vi "SVN Master Method Checkout.vi"(8 "error in (no error)":errorcluster, 11 "Method Name":string) -> (0 "error out":errorcluster, 1 "Method Version":i32, 2 "versions":i32[](array[numeric]), 3 "Method Names":string[](array[string]), 4 "Method Exists":bool, 6 "method version folder":path)   [LabVIEW 2012]
uses:
  Folders.ctl
  ReadWrite.ctl
  Which method type.ctl
  Design Server.lvlib
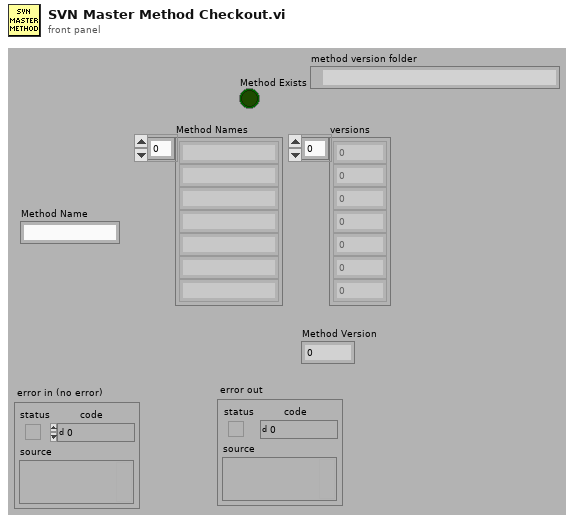
[diagram p1: front panel]
types:
  T1 = typedef "Design Server.lvlib/Folders.ctl" = enum16{"MathcadMethods", "RequestedDesigns", "CompletedDesigns", "MathcadCode", "CollabnetSVN.exe"}
  T2 = typedef "ReadWrite.ctl" = enum16{"Read", "Write"}
  T3 = typedef "Which method type.ctl" = enum16{"Master Method", "Method"}
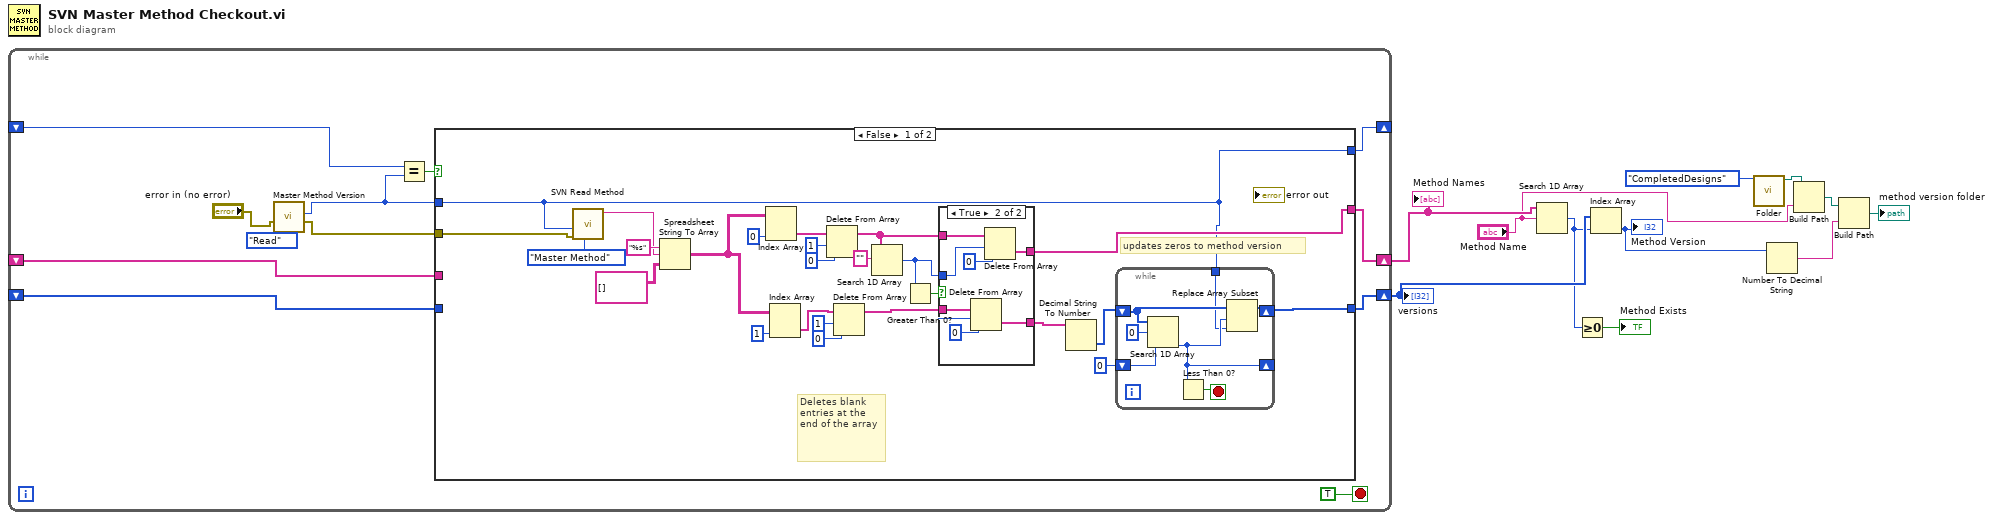
[diagram p0: block diagram]
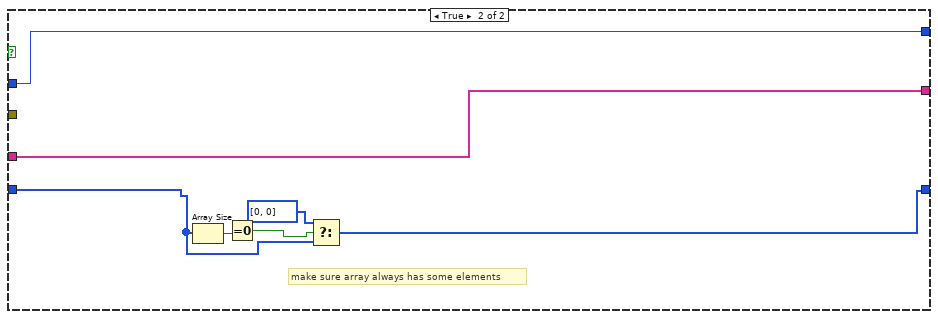
[diagram p3: hidden frame]
diagram:
  n1 = while {
    shift-right: [w20] -> _
    shift-left: _ -> [w22]
    shift-right: [w19] -> w11
    shift-left: _ -> [w17]
    shift-right: [w18] -> w10
    shift-left: _ -> [w16]
    stop <- TRUE stop-if-true
    n2 = call "Master Method Version.vi"("Config"=ReadWrite."Read", "error in (no error)"="error in (no error)") -> ("error out"=w13:errorcluster, "Current Master Method Version"=w12:i32)  [unwired: 6 in, 2 out]
    n3 = Equal?(x=w22, y=w12) -> (x = y?=w21:bool)
    n4 = case shown="False" w21 {
      tunnel: w12 -> [w25 w70]
      tunnel: [w25 w70] -> w20
      tunnel: [w27 w65] -> w18
      tunnel: [w26 w71] -> w19
      tunnel: w17 -> [_ w71]
      tunnel: w16 -> [_ w66]
      tunnel: w13 -> [w24 _]
      frame False {
        # "updates zeros to method version"
        # "Deletes blank entries at the end of the array"
        n5 = call "SVN Read Method.vi"("Which Method Type"=Which_method_type."Master Method", "error in (no error)"=w24, "Method version"=w25) -> ("Method text"=w29:string)  [unwired: 6 in, 2 out]
        n6 = Spreadsheet String To Array(format string="%s", spreadsheet string=w29, array type (2D Dbl)=string[][] []) -> (array=w34:string[][])  [unwired: 1 in]
        n7 = Index Array(array=w34, index (col)=0 ("index")) -> (element=w43:string[])  [unwired: 1 in]
        n8 = Index Array(array=w34, index (col)=1 ("index")) -> (element=w37:string[])  [unwired: 1 in]
        n9 = Delete From Array(array=w43, length=1, index=0) -> (array with subset deleted=w41:string[])  [unwired: 1 out]
        n10 = Delete From Array(array=w37, length=1, index=0) -> (array with subset deleted=w36:string[])  [unwired: 1 out]
        n11 = Search 1D Array(1D array=w41, element="") -> (index of element=w30:i32)  [unwired: 1 in]
        n12 = Greater Than 0?(x=w30) -> (x > 0?=w31:bool)
        n13 = case shown="True" w31 {
          tunnel: w41 -> [w50 w56]
          tunnel: w36 -> [w49 w54]
          tunnel: [w49 w53] -> w35
          tunnel: w30 -> [_ w52]
          tunnel: [w50 w51] -> w26
          frame False {
          }
          frame True {
            n14 = Delete From Array(array=w54, length=w52, index=0) -> (deleted portion=w53:string[])  [unwired: 1 out]
            n15 = Delete From Array(array=w56, length=w52, index=0) -> (deleted portion=w51:string[])  [unwired: 1 out]
          }
        }
        n16 = Decimal String To Number(string=w35) -> (number=w32:i32[])  [unwired: 2 in, 1 out]
        n17 = while {
          shift-right: [w62] -> _
          shift-left: 0 ("index of element") -> [w64]
          shift-right: [w61] -> w27
          shift-left: w32 -> [w60]
          tunnel: w25 -> [w58]
          stop <- w63 stop-if-true
          n18 = Search 1D Array(1D array=w60, element=0, start index (0)=w64) -> (index of element=w62:i32)
          n19 = Less Than 0?(x=w62) -> (x < 0?=w63:bool)
          n20 = Replace Array Subset(array=w60, new element=w58, index=w62) -> (w61:i32[])
        }
      }
      frame True {
        # "make sure array always has some elements"
        n21 = Array Size(array=w66) -> (size(s)=w69:i32)
        n22 = Equal To 0?(x=w69) -> (x = 0?=w67:bool)
        n23 = Select(t=i32[] [0, 0], s=w67, f=w66) -> (s? t:f=w65:i32[])
      }
    }
  }
  "Method Names" <- w11
  "versions" <- w10
  n24 = Search 1D Array(1D array=w11, element="Method Name") -> (index of element=w9:i32)  [unwired: 1 in]
  n25 = Greater Or Equal To 0?(x=w9) -> (x >= 0?=→"Method Exists":bool)
  n26 = Index Array(array=w10, index=w9) -> (element=w4:i32)
  "Method Version" <- w4
  n27 = call "Folder.vi"("Folders"=Folders."CompletedDesigns") -> ("FolderPath"=w7:path)  [unwired: 8 in, 2 out]
  n28 = Number To Decimal String(number=w4) -> (decimal integer string=w3:string)  [unwired: 1 in]
  n29 = Build Path(base path=w7, name or relative path="Method Name") -> (appended path=w6:path)
  n30 = Build Path(base path=w6, name or relative path=w3) -> (appended path=→"method version folder":path)
